vi "CTRE_Phoenix_MotorControl_ConfigAllCustomParameters.vi"(6 "timeoutMs":i32=50, 7 "Force Write":bool, 10 "CustomParam":T6, 11 "PhoenixMotorControlDevRef in":T1) -> (0 "AnyConfigFailed":bool, 3 "PhoenixMotorControlDevRef out":T1)   [LabVIEW 2017]
uses:
  <vilib>/Rock Robotics/WPI/ThirdParty/Phoenix-LabVIEW/Controls/CTRE_Phoenix_CustomParamConfiguration.ctl
  <vilib>/Rock Robotics/WPI/MotorControl/WPI_MotorControlDeviceRef.ctl
  <vilib>/Rock Robotics/WPI/MotorControl/WPI_MotorControlType.ctl
  <vilib>/Rock Robotics/SystemInterfaces/DIO/FPGA_DIOPWMChannel.ctl
  <vilib>/Rock Robotics/WPI/PWM/WPI_PWMDeadband.ctl
  <vilib>/Rock Robotics/SystemInterfaces/DIO/FPGA_DIOChannel.ctl
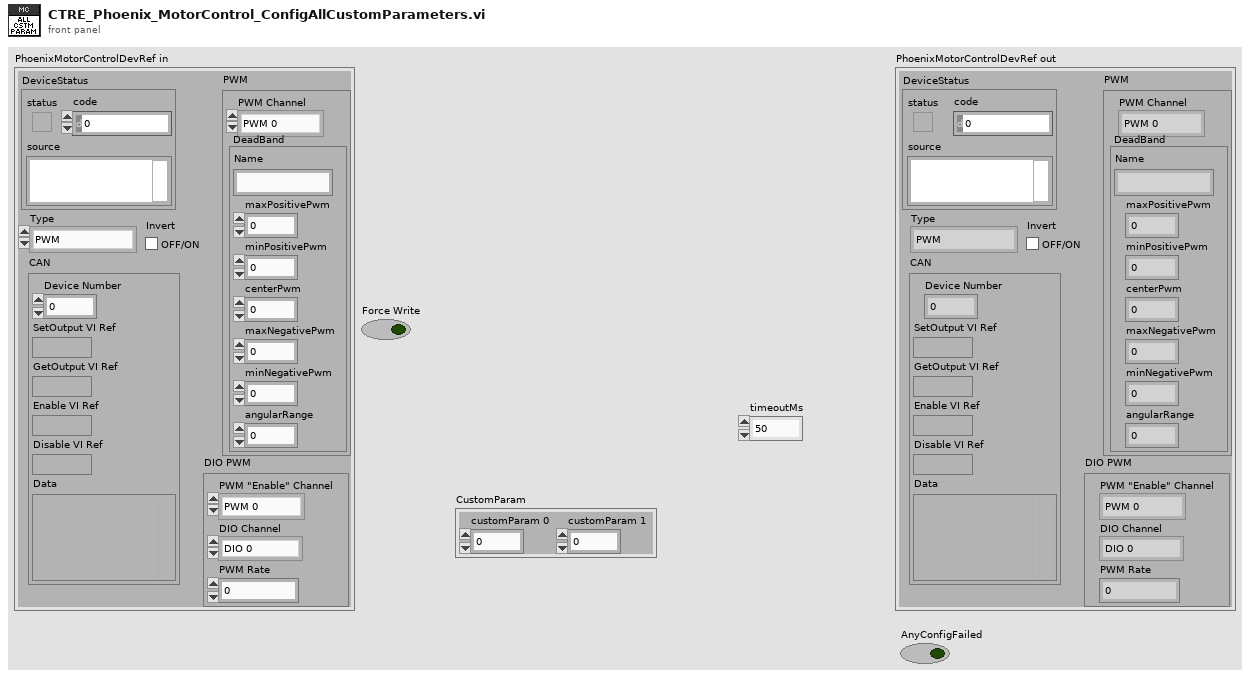
[diagram p1: front panel]
types:
  T1 = typedef "WPI_MotorControlDeviceRef.ctl" = cluster{"DeviceStatus":errorcluster, "Type":T2, "PWM":cluster{"PWM Channel":T3, "DeadBand":T4}, "CAN":cluster{"Device Number":u8, "SetOutput VI Ref":variant, "GetOutput VI Ref":variant, "Enable VI Ref":variant, "Disable VI Ref":variant, "Data":variant}, "Invert":bool, "DIO PWM":cluster{"PWM \"Enable\" Channel":T3, "DIOChannel":T5, "PWM Rate":dbl}}
  T2 = typedef "WPI_MotorControlType.ctl" = enum16{"PWM", "CAN", "DIO PWM"}
  T3 = typedef "FPGA_DIOPWMChannel.ctl" = enum8{"PWM 0", "PWM 1", "PWM 2", "PWM 3", "PWM 4", "PWM 5", "PWM 6", "PWM 7", "PWM 8", "PWM 9", "PWM MXP 0", "PWM MXP 1", "PWM MXP 2", "PWM MXP 3", "PWM MXP 4", "PWM MXP 5", "PWM MXP 6", "PWM MXP 7", "PWM MXP 8", "PWM MXP 9", "Invalid"}
  T4 = typedef "WPI_PWMDeadband.ctl" = cluster{"Name":string, "maxPositivePwm":i32, "minPositivePwm":i32, "centerPwm":i32, "maxNegativePwm":i32, "minNegativePwm":i32, "angularRange":u16}
  T5 = typedef "FPGA_DIOChannel.ctl" = enum8{"DIO 0", "DIO 1", "DIO 2", "DIO 3", "DIO 4", "DIO 5", "DIO 6", "DIO 7", "DIO 8", "DIO 9", "DIO MXP 0", "DIO MXP 1", "DIO MXP 2", "DIO MXP 3", "DIO MXP 4", "DIO MXP 5", "DIO MXP 6", "DIO MXP 7", "DIO MXP 8", "DIO MXP 9", "DIO MXP 10", "DIO MXP 11", "DIO MXP 12", "DIO MXP 13", "DIO MXP 14", "DIO MXP 15", "SPI Port CS1", "SPI Port CS2", "SPI Port CS3", "SPI Port MISO", "SPI Port MOSI", "Invalid"}
  T6 = typedef "CTRE_Phoenix_CustomParamConfiguration.ctl" = cluster{"customParam 0":i32, "customParam 1":i32}
  T7 = cluster{"customParam 0":bool, "customParam 1":bool}
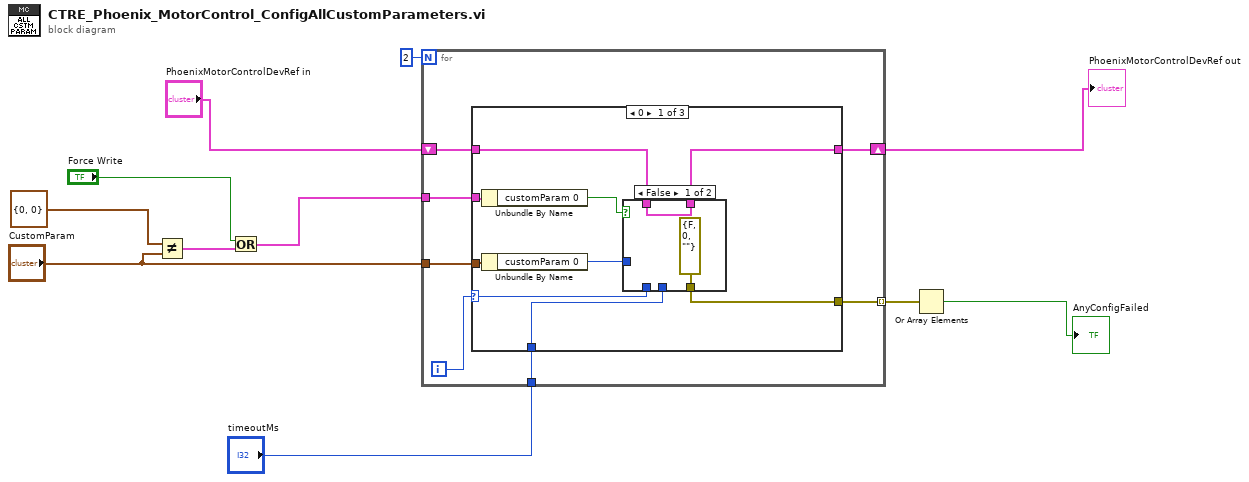
[diagram p0: block diagram]
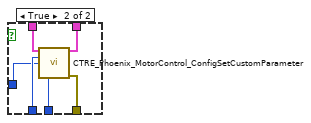
[diagram p2: hidden frame]
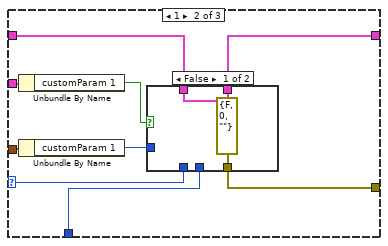
[diagram p3: hidden frame]
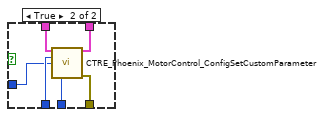
[diagram p4: hidden frame]
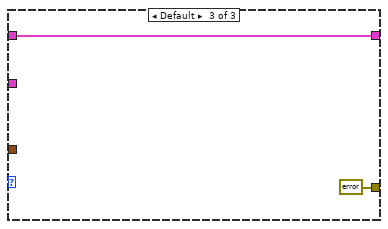
[diagram p5: hidden frame]
diagram:
  n1 = Not Equal?(x=T6 {"customParam 0"=0, "customParam 1"=0}, y="CustomParam") -> (x != y?=w3:T7)
  n2 = Or(x="Force Write", y=w3) -> (x .or. y?=w1:T7)
  n3 = for {
    N: 2 -> [_]
    tunnel: "CustomParam" -> [w17]
    shift-right: [w15] -> w9
    shift-left: "PhoenixMotorControlDevRef in" -> [w16]
    tunnel: "timeoutMs" -> [w14]
    tunnel: [w13] -> w7 mode=indexing
    tunnel: w1 -> [w12]
    i -> [w18]
    n4 = case shown="0" w18 {
      selector: w18 -> [w25 w42 _]
      tunnel: w17 -> [w24 w41 _]
      tunnel: w16 -> [w27 w44 w54]
      tunnel: [w26 w43 w54] -> w15
      tunnel: w14 -> [w22 w39 _]
      tunnel: [w21 w38 errorcluster {"status"=FALSE, "code"=0, "source"=""} ("error out")] -> w13
      tunnel: w12 -> [w20 w37 _]
      frame 0 {
        n5 = Unbundle By Name(w20) -> ("customParam 0"=w19:bool)
        n6 = Unbundle By Name(w24) -> ("customParam 0"=w23:i32)
        n7 = case shown="False" w19 {
          tunnel: w27 -> [w29 w35]
          tunnel: [w29 w34] -> w26
          tunnel: w25 -> [_ w33]
          tunnel: w23 -> [_ w32]
          tunnel: w22 -> [_ w31]
          tunnel: [errorcluster {"status"=FALSE, "code"=0, "source"=""} ("error out") w30] -> w21
          frame False {
          }
          frame True {
            n8 = call <vilib>:"CTRE_Phoenix_MotorControl_ConfigSetCustomParameter.vi"("PhoenixMotorControlDevRef"=w35, "paramIdx"=w33, "value"=w32, "timeoutMs"=w31) -> ("PhoenixMotorControlDevRef"=w34:T1, "error out"=w30:errorcluster)  [unwired: 10 in]
          }
        }
      }
      frame 1 {
        n9 = Unbundle By Name(w37) -> ("customParam 1"=w36:bool)
        n10 = Unbundle By Name(w41) -> ("customParam 1"=w40:i32)
        n11 = case shown="False" w36 {
          tunnel: w44 -> [w46 w52]
          tunnel: [w46 w51] -> w43
          tunnel: w42 -> [_ w50]
          tunnel: w40 -> [_ w49]
          tunnel: w39 -> [_ w48]
          tunnel: [errorcluster {"status"=FALSE, "code"=0, "source"=""} ("error out") w47] -> w38
          frame False {
          }
          frame True {
            n12 = call <vilib>:"CTRE_Phoenix_MotorControl_ConfigSetCustomParameter.vi"("PhoenixMotorControlDevRef"=w52, "paramIdx"=w50, "value"=w49, "timeoutMs"=w48) -> ("PhoenixMotorControlDevRef"=w51:T1, "error out"=w47:errorcluster)  [unwired: 10 in]
          }
        }
      }
      frame Default {
      }
    }
  }
  "PhoenixMotorControlDevRef out" <- w9
  n13 = Or Array Elements(Boolean array=w7) -> (logical OR=→"AnyConfigFailed":bool)
